vi "Application Control View.vi"(0 "Model in":refnum<class "Model.lvclass">) -> ()   [LabVIEW 2016, in "M1M3SupportEUI_Views.lvlib"]
uses:
  M1M3SupportEUI_Views.lvlib
  Model/Model.lvclass
  M1M3 Support Events/M1M3 Support Events.lvclass/M1M3 Support Events.ctl
  SALLV_m1m3/DataTypes/command_Start.ctl
  SALLV_m1m3/DataTypes/command_Standby.ctl
  SALLV_m1m3/DataTypes/command_Shutdown.ctl
  SALLV_m1m3/DataTypes/command_Enable.ctl
  SALLV_m1m3/DataTypes/command_Disable.ctl
  SALLV_m1m3/DataTypes/command_EnterEngineering.ctl
  SALLV_m1m3/DataTypes/command_ExitEngineering.ctl
  SALLV_m1m3/DataTypes/command_RaiseM1M3.ctl
  SALLV_m1m3/DataTypes/command_AbortRaiseM1M3.ctl
  SALLV_m1m3/DataTypes/command_LowerM1M3.ctl
  M1M3 Support Events/M1M3 Support Events.lvclass
  SALLV_m1m3/SALLV_m1m3.lvlib
  EUI Events/EUI Events.lvclass
panel:
  in  "AbortRaiseMirror IsTrue":bool
  in  "LowerMirror IsTrue":bool
  in  "ExitEngineering IsTrue":bool
  in  "RaiseMirror IsTrue":bool
  in  "EnterEngineering IsTrue":bool
  in  "disableIsTrue":bool
  in  "enableIsTrue":bool
  in  "standbyIsTrue":bool
  in  "shutdownIsTrue":bool
  in  "startIsTrue":bool
types:
  T1 = typedef "M1M3SupportEUI_TypeDefs.lvlib/M1M3 Support Events.ctl" = cluster{"Inclinometer  Data":refnum<user-event>, "IMS Data":refnum<user-event>, "SAL Connected":refnum<user-event>, "Accelerometer Data":refnum<user-event>, "OuterLoop Data":refnum<user-event>, "ErrorCode Event":refnum<user-event>, "InterlockStatus Event":refnum<user-event>, "InterlockWarning Event":refnum<user-event>, "Gyro Data":refnum<user-event>, "HP Actuator Info Event":refnum<user-event>, " FA Info Event":refnum<user-event>, "HP Monitor Info Event":refnum<user-event>, "FA Data":refnum<user-event>, "HP Actuator data":refnum<user-event>, "HP Monitor data":refnum<user-event>, "Air Supply Status Event":refnum<user-event>, "Air Supply Warning Event":refnum<user-event>, "Power Data":refnum<user-event>, "PID Data":refnum<user-event>, "PID Info Event":refnum<user-event>, "Power Status Event":refnum<user-event>, "Power Supply Status Event":refnum<user-event>, "Power Warning Event":refnum<user-event>, "Summary State Event":refnum<user-event>, "Detailed State Event":refnum<user-event>, "FA Force Warning Event":refnum<user-event>, "FA Warning Event":refnum<user-event>, "FA State Event":refnum<user-event>, "Applied AberrationForces Event":refnum<user-event>, "Applied Acceleration Forcces Event":refnum<user-event>, "Applied Azimuth Forces Event":refnum<user-event>, "Applied Active Optic Forces Event":refnum<user-event>, "Applied Balance Forces Event":refnum<user-event>, "Applied Cylinder Forces Event":refnum<user-event>, "Applied Elevation Forces Event":refnum<user-event>, "Applied Forces Event":refnum<user-event>, "Applied Offset Forces Event":refnum<user-event>, "Applied Static Forces Event":refnum<user-event>, "Applied Thermal Forces Event":refnum<user-event>, "Applied Velocity Forces Event":refnum<user-event>, "Rejected Aberration Force Event":refnum<user-event>, "Rejected Acceleration Forces Event":refnum<user-event>, "Rejected Active Optic Forces Event":refnum<user-event>, "Rejected Azimuth Forces Event":refnum<user-event>, "Rejected Balance Forces Event":refnum<user-event>, "Rejected Cylinder Forces Event":refnum<user-event>, "Rejected Elevation Forces Event":refnum<user-event>, "Rejected Forces Event":refnum<user-event>, "Rejected Offset Forces Event":refnum<user-event>, "Rejected Static Forces Event":refnum<user-event>, "Rejected Thermal Forces Event":refnum<user-event>, "Rejected Velocity Forces Event":refnum<user-event>, "Command Rejection Event":refnum<user-event>, "Setting Verions Event":refnum<user-event>, "Settings Applied Event":refnum<user-event>, "HP Actuator State Event":refnum<user-event>, "HP Actuator Warning Event":refnum<user-event>, "HP Monitor State Event":refnum<user-event>, "HP Monitor Warning Event":refnum<user-event>, "Accelerometer Warning Event":refnum<user-event>, "Applied Settings Match Start Event":refnum<user-event>, "Cell Light Status Event ":refnum<user-event>, "Cell Light Warning Event":refnum<user-event>, "Displacement Sensor Warning Event":refnum<user-event>, "Force Setpoint Warning Event":refnum<user-event>, "Gyro Warning Event ":refnum<user-event>, "ILC Warning Event ":refnum<user-event>, "Inclinometer Sensor Warning Event ":refnum<user-event>}
  T2 = enum16{"", "DetailedState_DetailedStates_DisabledState", "DetailedState_DetailedStates_EnabledState", "DetailedState_DetailedStates_FaultState", "DetailedState_DetailedStates_OfflineState", "DetailedState_DetailedStates_StandbyState", "DetailedState_DetailedStates_ParkedState", "DetailedState_DetailedStates_RaisingState", "DetailedState_DetailedStates_ActiveState", "DetailedState_DetailedStates_LoweringState", "DetailedState_DetailedStates_EngineeringState", "DetailedState_DetailedStates_ParkedEngineeringState", "DetailedState_DetailedStates_RaisingEngineeringState", "DetailedState_DetailedStates_ActiveEngineeringState", "DetailedState_DetailedStates_LoweringEngineeringState", "DetailedState_DetailedStates_LoweringFaultState", "DetailedState_DetailedStates_ProfileHardpointCorrectionState"}
  T3 = typedef "SALLV_m1m3.lvlib/command_Start.ctl" = cluster{"Start":bool, "SettingsToApply":string}
  T4 = typedef "SALLV_m1m3.lvlib/command_Standby.ctl" = cluster{"Standby":bool}
  T5 = typedef "SALLV_m1m3.lvlib/command_Shutdown.ctl" = cluster{"Shutdown":bool}
  T6 = typedef "SALLV_m1m3.lvlib/command_Enable.ctl" = cluster{"Enable":bool}
  T7 = typedef "SALLV_m1m3.lvlib/command_Disable.ctl" = cluster{"Disable":bool}
  T8 = typedef "SALLV_m1m3.lvlib/command_EnterEngineering.ctl" = cluster{"EnterEngineering":bool}
  T9 = typedef "SALLV_m1m3.lvlib/command_ExitEngineering.ctl" = cluster{"ExitEngineering":bool}
  T10 = typedef "SALLV_m1m3.lvlib/command_RaiseM1M3.ctl" = cluster{"RaiseM1M3":bool, "BypassReferencePosition":bool}
  T11 = typedef "SALLV_m1m3.lvlib/command_AbortRaiseM1M3.ctl" = cluster{"AbortRaiseM1M3":bool}
  T12 = typedef "SALLV_m1m3.lvlib/command_LowerM1M3.ctl" = cluster{"LowerM1M3":bool}
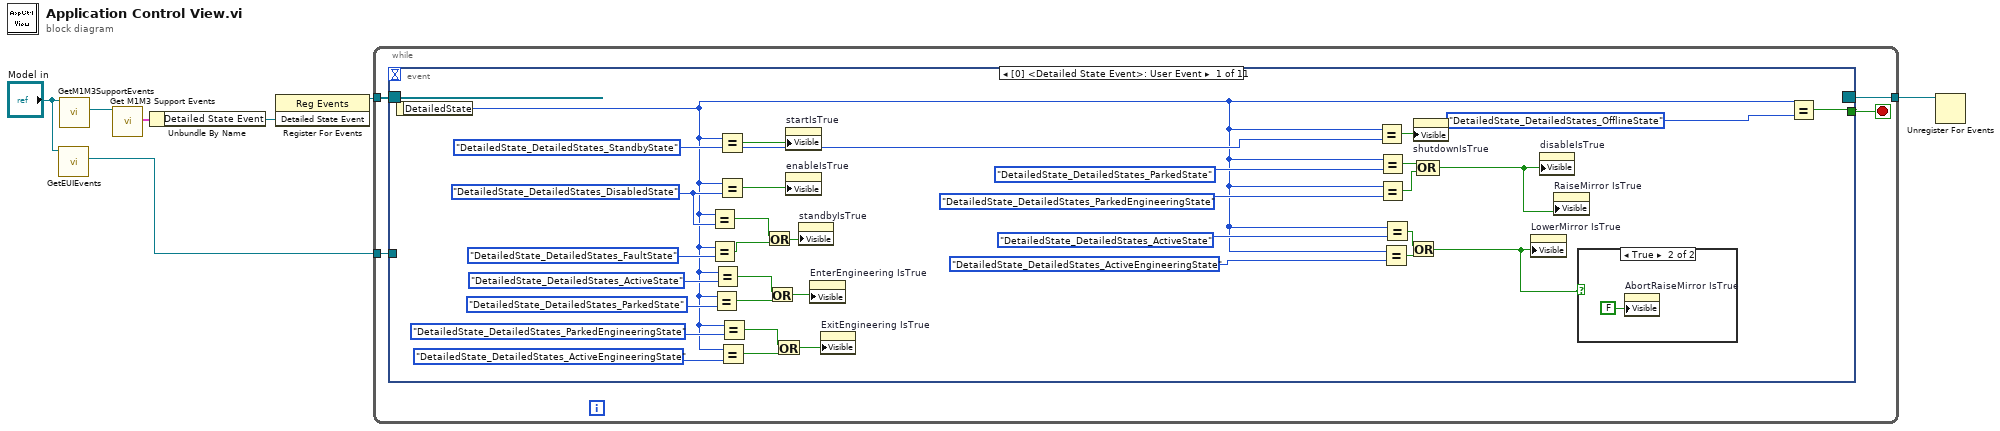
[diagram p0: block diagram]
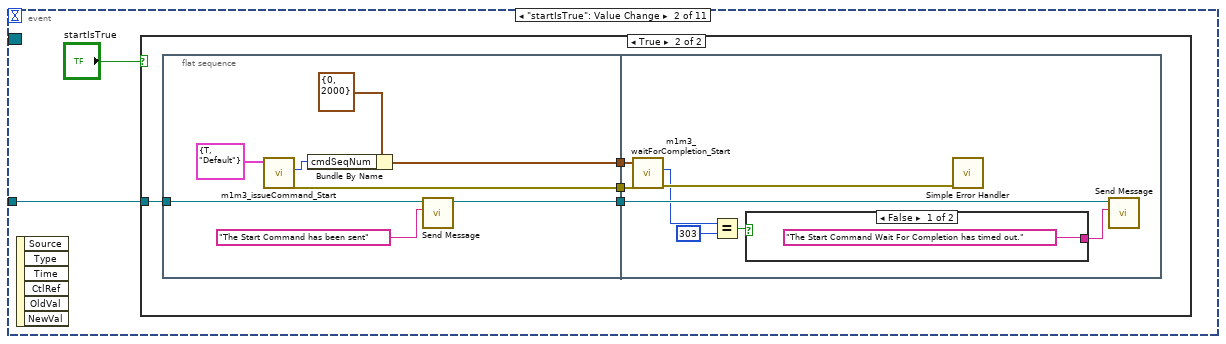
[diagram p3: hidden frame]
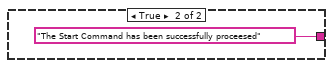
[diagram p5: hidden frame]
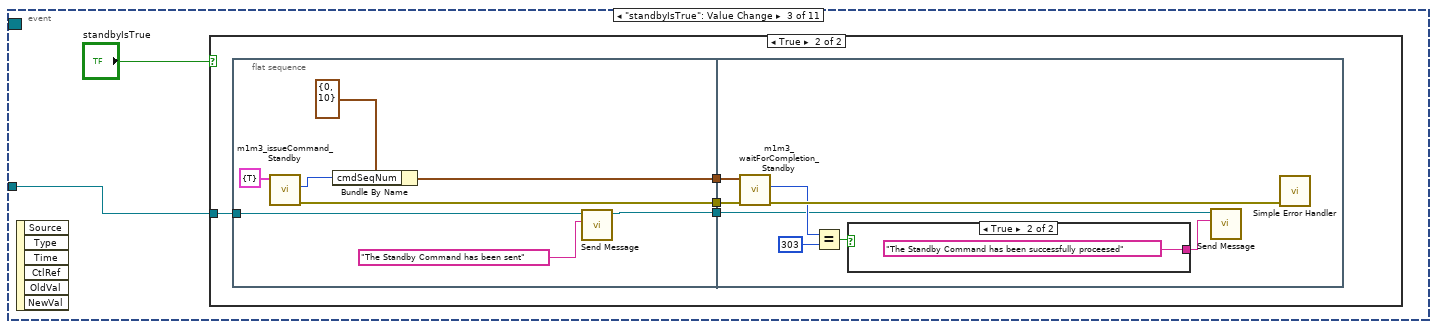
[diagram p6: hidden frame]
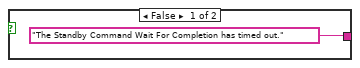
[diagram p8: hidden frame]
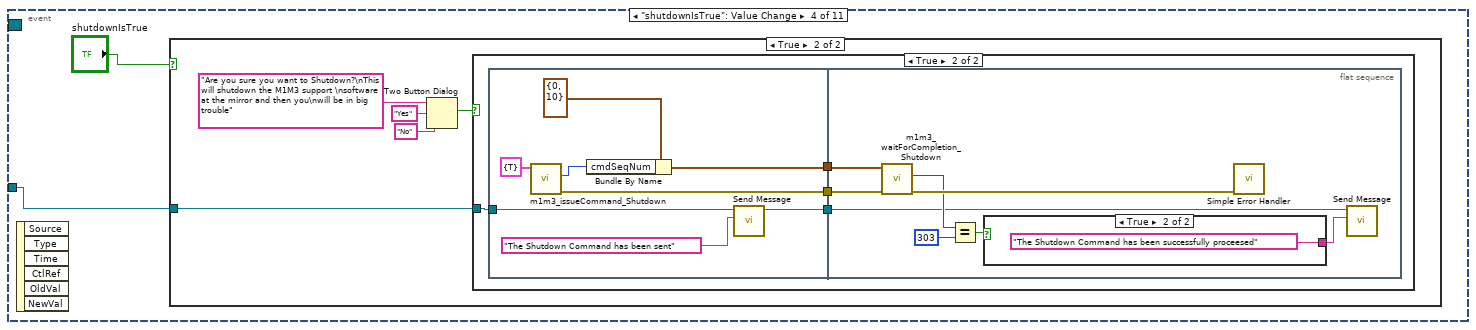
[diagram p9: hidden frame]
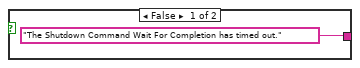
[diagram p12: hidden frame]
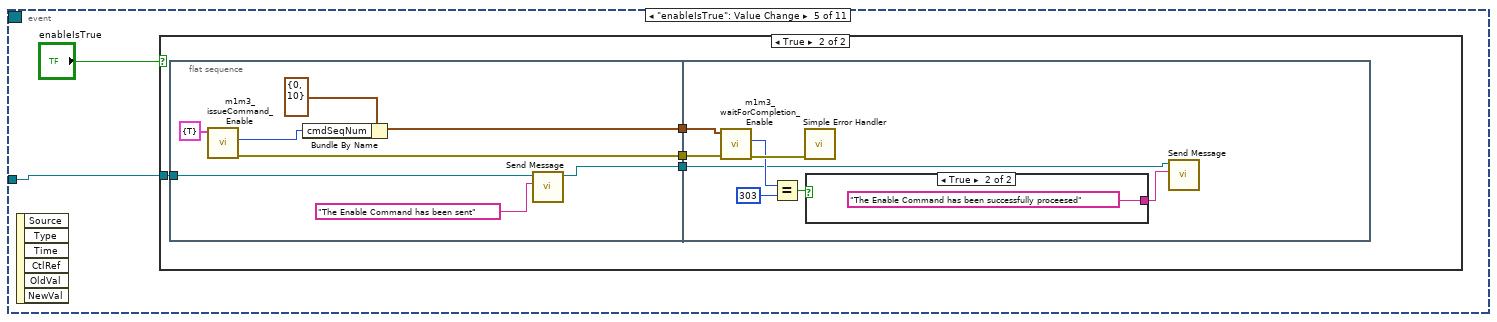
[diagram p13: hidden frame]
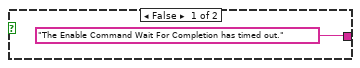
[diagram p15: hidden frame]
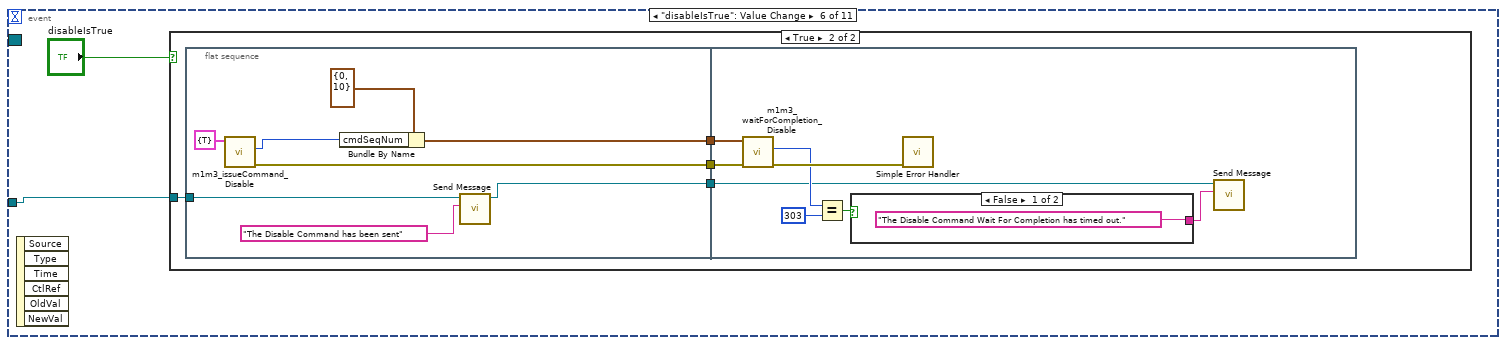
[diagram p16: hidden frame]
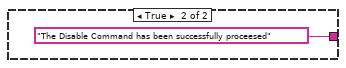
[diagram p18: hidden frame]
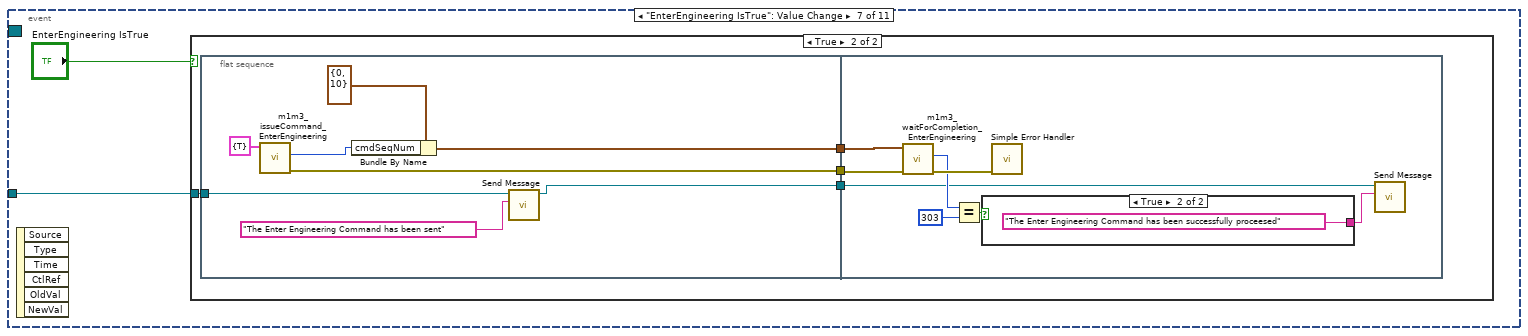
[diagram p19: hidden frame]
diagram:
  n1 = call "GetEUIEvents.vi"("Model in"="Model in") -> ("EUI Events out"=w1:refnum<class "EUI Events.lvclass">)  [unwired: 8 in, 2 out]
  n2 = call "GetM1M3SupportEvents.vi"("Model in"="Model in") -> ("M1M3 Support Events out"=w3:refnum<class "M1M3 Support Events.lvclass">)  [unwired: 8 in, 2 out]
  n3 = call "Get M1M3 Support Events.vi"("M1M3 Support Events in"=w3) -> ("M1M3 Support Events"=w6:T1)  [unwired: 9 in, 1 out]
  n4 = Unbundle By Name(w6) -> ("Detailed State Event"=w5:refnum<user-event>)
  n5 = register-events(w5) -> (reference out=w7:refnum<event-registration>)  [unwired: 2 in, 1 out]
  n6 = while {
    tunnel: w7 -> [w11]
    tunnel: [w10] -> w4
    tunnel: w1 -> [w8]
    stop <- w9 stop-if-true
    n7 = event shown="[0] <Detailed State Event>: User Event" {
      selector: w11 -> [_ _ _ _ _ _ _ _ _ _ _]
      dyn-events: [_ _ _ _ _ _ _ _ _ _ _] -> w10
      timeout: _ -> [_ _ _ _ _ _ _ _ _ _ _]
      tunnel: [w43 _ _ _ _ _ _ _ _ _ _] -> w9
      tunnel: w8 -> [_ w45 w69 w93 w122 w146 w170 w194 w218 w243 w267]
      event User Event {
        w26 = T2."DetailedState_DetailedStates_DisabledState" ("y")
        w20 = T2."DetailedState_DetailedStates_StandbyState" ("y")
        n8 = event-data() -> ("DetailedState"=w13:T2)  [unwired: 1 in]
        n9 = Equal?(x=w13, y=w26) -> (x = y?=w39:bool)
        n10 = Equal?(x=w13, y=T2."DetailedState_DetailedStates_FaultState") -> (x = y?=w40:bool)
        n11 = Equal?(x=w13, y=T2."DetailedState_DetailedStates_ParkedState") -> (x = y?=w35:bool)
        n12 = Equal?(x=w13, y=T2."DetailedState_DetailedStates_ActiveState") -> (x = y?=w36:bool)
        n13 = Equal?(x=w13, y=w20) -> (x = y?=w42:bool)
        n14 = Equal?(x=w13, y=w26) -> (x = y?=w41:bool)
        n15 = Equal?(x=w13, y=T2."DetailedState_DetailedStates_ActiveEngineeringState") -> (x = y?=w33:bool)
        n16 = Equal?(x=w13, y=T2."DetailedState_DetailedStates_ParkedEngineeringState") -> (x = y?=w32:bool)
        n17 = Or(x=w39, y=w40) -> (x .or. y?=w38:bool)
        n18 = Or(x=w36, y=w35) -> (x .or. y?=w34:bool)
        n19 = Or(x=w32, y=w33) -> (x .or. y?=w31:bool)
        n20 = property on="startIsTrue" class="Bool"("Visible"=w42) -> ()  [unwired: 2 in, 2 out]
        n21 = property on="enableIsTrue" class="Bool"("Visible"=w41) -> ()  [unwired: 2 in, 2 out]
        n22 = property on="standbyIsTrue" class="Bool"("Visible"=w38) -> ()  [unwired: 2 in, 2 out]
        n23 = property on="EnterEngineering IsTrue" class="Bool"("Visible"=w34) -> ()  [unwired: 2 in, 2 out]
        n24 = property on="ExitEngineering IsTrue" class="Bool"("Visible"=w31) -> ()  [unwired: 2 in, 2 out]
        n25 = Equal?(x=w13, y=w20) -> (x = y?=w37:bool)
        n26 = Equal?(x=w13, y=T2."DetailedState_DetailedStates_ParkedState") -> (x = y?=w28:bool)
        n27 = Equal?(x=w13, y=T2."DetailedState_DetailedStates_ParkedEngineeringState") -> (x = y?=w27:bool)
        n28 = Equal?(x=w13, y=T2."DetailedState_DetailedStates_ActiveEngineeringState") -> (x = y?=w29:bool)
        n29 = Equal?(x=w13, y=T2."DetailedState_DetailedStates_ActiveState") -> (x = y?=w30:bool)
        n30 = Or(x=w30, y=w29) -> (x .or. y?=w12:bool)
        n31 = property on="shutdownIsTrue" class="Bool"("Visible"=w37) -> ()  [unwired: 2 in, 2 out]
        n32 = Compound Arithmetic op=OR(w28, w27) -> (w17:bool)
        n33 = property on="LowerMirror IsTrue" class="Bool"("Visible"=w12) -> ()  [unwired: 2 in, 2 out]
        n34 = property on="disableIsTrue" class="Bool"("Visible"=w17) -> ()  [unwired: 2 in, 2 out]
        n35 = property on="RaiseMirror IsTrue" class="Bool"("Visible"=w17) -> ()  [unwired: 2 in, 2 out]
        n36 = case shown="True" w12 {
          frame False {
          }
          frame True {
            n37 = property on="AbortRaiseMirror IsTrue" class="Bool"("Visible"=FALSE) -> ()  [unwired: 2 in, 2 out]
          }
        }
        n38 = Equal?(x=w13, y=T2."DetailedState_DetailedStates_OfflineState") -> (x = y?=w43:bool)
      }
      event "startIsTrue": Value Change {
        n39 = event-data() -> ()  [unwired: 1 in, 6 out]
        n40 = case shown="True" "startIsTrue" {
          tunnel: w45 -> [_ w48]
          frame False {
          }
          frame True {
            n41 = flat-sequence {
              tunnel: [w57] -> w50
              tunnel: [w54] -> w49
              tunnel: w48 -> [w53]
              tunnel: [w51] -> w47
              tunnel: w50 -> [w65]
              tunnel: w49 -> [w66]
              tunnel: w47 -> [w63]
              frame #0 {
                n42 = call "m1m3_issueCommand_Start.vi"("command_Start_Ctl"=T3 {"Start"=TRUE, "SettingsToApply"="Default"}) -> ("error out"=w57:errorcluster, "function return"=w55:i32)  [unwired: 8 in, 1 out]
                n43 = Bundle By Name(cluster=cluster{"cmdSeqNum":i32, "timeout":u32} {"cmdSeqNum"=0, "timeout"=2000} ("waitComplete_Ctl"), "cmdSeqNum"=w55) -> (w54:cluster{"cmdSeqNum":i32, "timeout":u32})
                n44 = call "Send Message.vi"("Message"="The Start Command has been sent", "EUI Events in"=w53) -> ("EUI Events out"=w51:refnum<class "EUI Events.lvclass">)  [unwired: 8 in, 1 out]
              }
              frame #1 {
                n45 = call "m1m3_waitForCompletion_Start.vi"("error in (no error)"=w65, "waitComplete_Ctl"=w66) -> ("error out"=w64:errorcluster, "function return"=w61:i32)  [unwired: 7 in, 1 out]
                n46 = Equal?(x=w61, y=303) -> (x = y?=w62:bool)
                n47 = case shown="False" w62 {
                  tunnel: ["The Start Command Wait For Completion has timed out." ("Message") "The Start Command has been successfully proceesed" ("Message")] -> w60
                  frame False {
                  }
                  frame True {
                  }
                }
                n48 = call <vilib>:"Simple Error Handler.vi"("error in (no error)"=w64) -> ()  [unwired: 4 in, 5 out]
                n49 = call "Send Message.vi"("Message"=w60, "EUI Events in"=w63) -> ()  [unwired: 8 in, 2 out]
              }
            }
          }
        }
      }
      event "standbyIsTrue": Value Change {
        n50 = event-data() -> ()  [unwired: 1 in, 6 out]
        n51 = case shown="True" "standbyIsTrue" {
          tunnel: w69 -> [_ w74]
          frame False {
          }
          frame True {
            n52 = flat-sequence {
              tunnel: w74 -> [w76]
              tunnel: [w81] -> w73
              tunnel: [w78] -> w72
              tunnel: [w75] -> w71
              tunnel: w73 -> [w88]
              tunnel: w72 -> [w89]
              tunnel: w71 -> [w83]
              frame #0 {
                n53 = call "m1m3_issueCommand_Standby.vi"("command_Standby_Ctl"=T4 {"Standby"=TRUE}) -> ("error out"=w81:errorcluster, "function return"=w79:i32)  [unwired: 8 in, 1 out]
                n54 = Bundle By Name(cluster=cluster{"cmdSeqNum":i32, "timeout":u32} {"cmdSeqNum"=0, "timeout"=10} ("waitComplete_Ctl"), "cmdSeqNum"=w79) -> (w78:cluster{"cmdSeqNum":i32, "timeout":u32})
                n55 = call "Send Message.vi"("Message"="The Standby Command has been sent", "EUI Events in"=w76) -> ("EUI Events out"=w75:refnum<class "EUI Events.lvclass">)  [unwired: 8 in, 1 out]
              }
              frame #1 {
                n56 = call "m1m3_waitForCompletion_Standby.vi"("error in (no error)"=w88, "waitComplete_Ctl"=w89) -> ("error out"=w90:errorcluster, "function return"=w84:i32)  [unwired: 7 in, 1 out]
                n57 = Equal?(x=w84, y=303) -> (x = y?=w86:bool)
                n58 = case shown="True" w86 {
                  tunnel: ["The Standby Command Wait For Completion has timed out." ("Message") "The Standby Command has been successfully proceesed" ("Message")] -> w87
                  frame False {
                  }
                  frame True {
                  }
                }
                n59 = call "Send Message.vi"("Message"=w87, "EUI Events in"=w83) -> ()  [unwired: 8 in, 2 out]
                n60 = call <vilib>:"Simple Error Handler.vi"("error in (no error)"=w90) -> ()  [unwired: 4 in, 5 out]
              }
            }
          }
        }
      }
      event "shutdownIsTrue": Value Change {
        n61 = event-data() -> ()  [unwired: 1 in, 6 out]
        n62 = case shown="True" "shutdownIsTrue" {
          tunnel: w93 -> [_ w95]
          frame False {
          }
          frame True {
            n63 = Two Button Dialog(message="Are you sure you want to Shutdown?\nThis will shutdown the M1M3 support \nsoftware at the mirror and then you\nwill be in big trouble", 1:"No" ("F button name (\"Cancel\")"), 2:"Yes" ("T button name (\"OK\")")) -> (T button?=w99:bool)
            n64 = case shown="True" w99 {
              tunnel: w95 -> [_ w101]
              frame False {
              }
              frame True {
                n65 = flat-sequence {
                  tunnel: [w108] -> w103
                  tunnel: [w107] -> w102
                  tunnel: w101 -> [w105]
                  tunnel: [w104] -> w100
                  tunnel: w103 -> [w118]
                  tunnel: w102 -> [w117]
                  tunnel: w100 -> [w112]
                  frame #0 {
                    n66 = call "m1m3_issueCommand_Shutdown.vi"("command_Shutdown_Ctl"=T5 {"Shutdown"=TRUE}) -> ("error out"=w107:errorcluster, "function return"=w110:i32)  [unwired: 8 in, 1 out]
                    n67 = Bundle By Name(cluster=cluster{"cmdSeqNum":i32, "timeout":u32} {"cmdSeqNum"=0, "timeout"=10} ("waitComplete_Ctl"), "cmdSeqNum"=w110) -> (w108:cluster{"cmdSeqNum":i32, "timeout":u32})
                    n68 = call "Send Message.vi"("Message"="The Shutdown Command has been sent", "EUI Events in"=w105) -> ("EUI Events out"=w104:refnum<class "EUI Events.lvclass">)  [unwired: 8 in, 1 out]
                  }
                  frame #1 {
                    n69 = call "m1m3_waitForCompletion_Shutdown.vi"("error in (no error)"=w117, "waitComplete_Ctl"=w118) -> ("error out"=w119:errorcluster, "function return"=w113:i32)  [unwired: 7 in, 1 out]
                    n70 = Equal?(x=w113, y=303) -> (x = y?=w115:bool)
                    n71 = case shown="True" w115 {
                      tunnel: ["The Shutdown Command Wait For Completion has timed out." ("Message") "The Shutdown Command has been successfully proceesed" ("Message")] -> w116
                      frame False {
                      }
                      frame True {
                      }
                    }
                    n72 = call <vilib>:"Simple Error Handler.vi"("error in (no error)"=w119) -> ()  [unwired: 4 in, 5 out]
                    n73 = call "Send Message.vi"("Message"=w116, "EUI Events in"=w112) -> ()  [unwired: 8 in, 2 out]
                  }
                }
              }
            }
          }
        }
      }
      event "enableIsTrue": Value Change {
        n74 = event-data() -> ()  [unwired: 1 in, 6 out]
        n75 = case shown="True" "enableIsTrue" {
          tunnel: w122 -> [_ w125]
          frame False {
          }
          frame True {
            n76 = flat-sequence {
              tunnel: [w132] -> w127
              tunnel: [w131] -> w126
              tunnel: w125 -> [w129]
              tunnel: [w128] -> w124
              tunnel: w127 -> [w142]
              tunnel: w126 -> [w141]
              tunnel: w124 -> [w136]
              frame #0 {
                n77 = call "m1m3_issueCommand_Enable.vi"("command_Enable_Ctl"=T6 {"Enable"=TRUE}) -> ("error out"=w131:errorcluster, "function return"=w133:i32)  [unwired: 8 in, 1 out]
                n78 = Bundle By Name(cluster=cluster{"cmdSeqNum":i32, "timeout":u32} {"cmdSeqNum"=0, "timeout"=10} ("waitComplete_Ctl"), "cmdSeqNum"=w133) -> (w132:cluster{"cmdSeqNum":i32, "timeout":u32})
                n79 = call "Send Message.vi"("Message"="The Enable Command has been sent", "EUI Events in"=w129) -> ("EUI Events out"=w128:refnum<class "EUI Events.lvclass">)  [unwired: 8 in, 1 out]
              }
              frame #1 {
                n80 = call "m1m3_waitForCompletion_Enable.vi"("error in (no error)"=w141, "waitComplete_Ctl"=w142) -> ("error out"=w143:errorcluster, "function return"=w137:i32)  [unwired: 7 in, 1 out]
                n81 = Equal?(x=w137, y=303) -> (x = y?=w139:bool)
                n82 = call <vilib>:"Simple Error Handler.vi"("error in (no error)"=w143) -> ()  [unwired: 4 in, 5 out]
                n83 = case shown="True" w139 {
                  tunnel: ["The Enable Command Wait For Completion has timed out." ("Message") "The Enable Command has been successfully proceesed" ("Message")] -> w140
                  frame False {
                  }
                  frame True {
                  }
                }
                n84 = call "Send Message.vi"("Message"=w140, "EUI Events in"=w136) -> ()  [unwired: 8 in, 2 out]
              }
            }
          }
        }
      }
      event "disableIsTrue": Value Change {
        n85 = event-data() -> ()  [unwired: 1 in, 6 out]
        n86 = case shown="True" "disableIsTrue" {
          tunnel: w146 -> [_ w151]
          frame False {
          }
          frame True {
            n87 = flat-sequence {
              tunnel: w151 -> [w155]
              tunnel: [w154] -> w150
              tunnel: [w153] -> w149
              tunnel: [w152] -> w148
              tunnel: w150 -> [w163]
              tunnel: w149 -> [w162]
              tunnel: w148 -> [w160]
              frame #0 {
                n88 = call "m1m3_issueCommand_Disable.vi"("command_Disable_Ctl"=T7 {"Disable"=TRUE}) -> ("error out"=w153:errorcluster, "function return"=w157:i32)  [unwired: 8 in, 1 out]
                n89 = Bundle By Name(cluster=cluster{"cmdSeqNum":i32, "timeout":u32} {"cmdSeqNum"=0, "timeout"=10} ("waitComplete_Ctl"), "cmdSeqNum"=w157) -> (w154:cluster{"cmdSeqNum":i32, "timeout":u32})
                n90 = call "Send Message.vi"("Message"="The Disable Command has been sent", "EUI Events in"=w155) -> ("EUI Events out"=w152:refnum<class "EUI Events.lvclass">)  [unwired: 8 in, 1 out]
              }
              frame #1 {
                n91 = call "m1m3_waitForCompletion_Disable.vi"("error in (no error)"=w162, "waitComplete_Ctl"=w163) -> ("error out"=w164:errorcluster, "function return"=w161:i32)  [unwired: 7 in, 1 out]
                n92 = Equal?(x=w161, y=303) -> (x = y?=w166:bool)
                n93 = case shown="False" w166 {
                  tunnel: ["The Disable Command Wait For Completion has timed out." ("Message") "The Disable Command has been successfully proceesed" ("Message")] -> w167
                  frame False {
                  }
                  frame True {
                  }
                }
                n94 = call <vilib>:"Simple Error Handler.vi"("error in (no error)"=w164) -> ()  [unwired: 4 in, 5 out]
                n95 = call "Send Message.vi"("Message"=w167, "EUI Events in"=w160) -> ()  [unwired: 8 in, 2 out]
              }
            }
          }
        }
      }
      event "EnterEngineering IsTrue": Value Change {
        n96 = event-data() -> ()  [unwired: 1 in, 6 out]
        n97 = case shown="True" "EnterEngineering IsTrue" {
          tunnel: w170 -> [_ w173]
          frame False {
          }
          frame True {
            n98 = flat-sequence {
              tunnel: [w180] -> w175
              tunnel: [w179] -> w174
              tunnel: w173 -> [w177]
              tunnel: [w176] -> w172
              tunnel: w175 -> [w190]
              tunnel: w174 -> [w189]
              tunnel: w172 -> [w184]
              frame #0 {
                n99 = call "m1m3_issueCommand_EnterEngineering.vi"("command_EnterEngineering_Ctl"=T8 {"EnterEngineering"=TRUE}) -> ("error out"=w179:errorcluster, "function return"=w181:i32)  [unwired: 8 in, 1 out]
                n100 = Bundle By Name(cluster=cluster{"cmdSeqNum":i32, "timeout":u32} {"cmdSeqNum"=0, "timeout"=10} ("waitComplete_Ctl"), "cmdSeqNum"=w181) -> (w180:cluster{"cmdSeqNum":i32, "timeout":u32})
                n101 = call "Send Message.vi"("Message"="The Enter Engineering Command has been sent", "EUI Events in"=w177) -> ("EUI Events out"=w176:refnum<class "EUI Events.lvclass">)  [unwired: 8 in, 1 out]
              }
              frame #1 {
                n102 = call "m1m3_waitForCompletion_EnterEngineering.vi"("error in (no error)"=w189, "waitComplete_Ctl"=w190) -> ("error out"=w191:errorcluster, "function return"=w185:i32)  [unwired: 7 in, 1 out]
                n103 = Equal?(x=w185, y=303) -> (x = y?=w187:bool)
                n104 = case shown="True" w187 {
                  tunnel: ["The Enter Engineering Command Wait For Completion has timed out." ("Message") "The Enter Engineering Command has been successfully proceesed" ("Message")] -> w188
                  frame False {
                  }
                  frame True {
                  }
                }
                n105 = call <vilib>:"Simple Error Handler.vi"("error in (no error)"=w191) -> ()  [unwired: 4 in, 5 out]
                n106 = call "Send Message.vi"("Message"=w188, "EUI Events in"=w184) -> ()  [unwired: 8 in, 2 out]
              }
            }
          }
        }
      }
      event "ExitEngineering IsTrue": Value Change {
        n107 = event-data() -> ()  [unwired: 1 in, 6 out]
        n108 = case shown="True" "ExitEngineering IsTrue" {
          tunnel: w194 -> [_ w197]
          frame False {
          }
          frame True {
            n109 = flat-sequence {
              tunnel: [w204] -> w199
              tunnel: [w203] -> w198
              tunnel: w197 -> [w201]
              tunnel: [w200] -> w196
              tunnel: w199 -> [w214]
              tunnel: w198 -> [w213]
              tunnel: w196 -> [w209]
              frame #0 {
                n110 = call "m1m3_issueCommand_ExitEngineering.vi"("command_ExitEngineering_Ctl"=T9 {"ExitEngineering"=TRUE}) -> ("error out"=w203:errorcluster, "function return"=w205:i32)  [unwired: 8 in, 1 out]
                n111 = Bundle By Name(cluster=cluster{"cmdSeqNum":i32, "timeout":u32} {"cmdSeqNum"=0, "timeout"=10} ("waitComplete_Ctl"), "cmdSeqNum"=w205) -> (w204:cluster{"cmdSeqNum":i32, "timeout":u32})
                n112 = call "Send Message.vi"("Message"="The Exit Engineering Command has been sent", "EUI Events in"=w201) -> ("EUI Events out"=w200:refnum<class "EUI Events.lvclass">)  [unwired: 8 in, 1 out]
              }
              frame #1 {
                n113 = call "m1m3_waitForCompletion_ExitEngineering.vi"("error in (no error)"=w213, "waitComplete_Ctl"=w214) -> ("error out"=w215:errorcluster, "function return"=w208:i32)  [unwired: 7 in, 1 out]
                n114 = Equal?(x=w208, y=303) -> (x = y?=w211:bool)
                n115 = call <vilib>:"Simple Error Handler.vi"("error in (no error)"=w215) -> ()  [unwired: 4 in, 5 out]
                n116 = case shown="True" w211 {
                  tunnel: ["The Exit Engineering Command Wait For Completion has timed out." ("Message") "The Exit Engineering Command has been successfully proceesed" ("Message")] -> w212
                  frame False {
                  }
                  frame True {
                  }
                }
                n117 = call "Send Message.vi"("Message"=w212, "EUI Events in"=w209) -> ()  [unwired: 8 in, 2 out]
              }
            }
          }
        }
      }
      event "RaiseMirror IsTrue": Value Change {
        n118 = event-data() -> ()  [unwired: 1 in, 6 out]
        n119 = case shown="True" "RaiseMirror IsTrue" {
          tunnel: w218 -> [_ w223]
          frame False {
          }
          frame True {
            n120 = flat-sequence {
              tunnel: w223 -> [w227]
              tunnel: [w226] -> w222
              tunnel: [w225] -> w221
              tunnel: [w224] -> w220
              tunnel: w222 -> [w237]
              tunnel: w221 -> [w235]
              tunnel: w220 -> [w234]
              frame #0 {
                n121 = call "m1m3_issueCommand_RaiseM1M3.vi"("command_RaiseM1M3_Ctl"=T10 {"RaiseM1M3"=TRUE, "BypassReferencePosition"=FALSE}) -> ("error out"=w224:errorcluster, "function return"=w230:i32)  [unwired: 8 in, 1 out]
                n122 = Bundle By Name(cluster=cluster{"cmdSeqNum":i32, "timeout":u32} {"cmdSeqNum"=0, "timeout"=10} ("waitComplete_Ctl"), "cmdSeqNum"=w230) -> (w225:cluster{"cmdSeqNum":i32, "timeout":u32})
                n123 = property on="AbortRaiseMirror IsTrue" class="Bool"("Visible"=TRUE) -> ()  [unwired: 2 in, 2 out]
                n124 = call "Send Message.vi"("Message"="The Raise Mirror Command has been sent", "EUI Events in"=w227) -> ("EUI Events out"=w226:refnum<class "EUI Events.lvclass">)  [unwired: 8 in, 1 out]
              }
              frame #1 {
                n125 = call "m1m3_waitForCompletion_RaiseM1M3.vi"("error in (no error)"=w234, "waitComplete_Ctl"=w235) -> ("error out"=w236:errorcluster, "function return"=w233:i32)  [unwired: 7 in, 1 out]
                n126 = Equal?(x=w233, y=303) -> (x = y?=w239:bool)
                n127 = case shown="False" w239 {
                  tunnel: ["The Raise Mirror Command Wait For Completion has timed out." ("Message") "The Raise Mirror Command has been successfully proceesed" ("Message")] -> w240
                  frame False {
                  }
                  frame True {
                  }
                }
                n128 = call <vilib>:"Simple Error Handler.vi"("error in (no error)"=w236) -> ()  [unwired: 4 in, 5 out]
                n129 = call "Send Message.vi"("Message"=w240, "EUI Events in"=w237) -> ()  [unwired: 8 in, 2 out]
              }
            }
          }
        }
      }
      event "AbortRaiseMirror IsTrue": Value Change {
        n130 = event-data() -> ()  [unwired: 1 in, 6 out]
        n131 = case shown="True" "AbortRaiseMirror IsTrue" {
          tunnel: w243 -> [_ w246]
          frame False {
          }
          frame True {
            n132 = flat-sequence {
              tunnel: [w253] -> w248
              tunnel: [w252] -> w247
              tunnel: w246 -> [w250]
              tunnel: [w249] -> w245
              tunnel: w248 -> [w263]
              tunnel: w247 -> [w262]
              tunnel: w245 -> [w258]
              frame #0 {
                n133 = call "m1m3_issueCommand_AbortRaiseM1M3.vi"("command_AbortRaiseM1M3_Ctl"=T11 {"AbortRaiseM1M3"=TRUE}) -> ("error out"=w252:errorcluster, "function return"=w254:i32)  [unwired: 8 in, 1 out]
                n134 = Bundle By Name(cluster=cluster{"cmdSeqNum":i32, "timeout":u32} {"cmdSeqNum"=0, "timeout"=10} ("waitComplete_Ctl"), "cmdSeqNum"=w254) -> (w253:cluster{"cmdSeqNum":i32, "timeout":u32})
                n135 = call "Send Message.vi"("Message"="The Abort Raise Mirror Command has been sent", "EUI Events in"=w250) -> ("EUI Events out"=w249:refnum<class "EUI Events.lvclass">)  [unwired: 8 in, 1 out]
              }
              frame #1 {
                n136 = call "m1m3_waitForCompletion_AbortRaiseM1M3.vi"("error in (no error)"=w262, "waitComplete_Ctl"=w263) -> ("error out"=w264:errorcluster, "function return"=w257:i32)  [unwired: 7 in, 1 out]
                n137 = Equal?(x=w257, y=303) -> (x = y?=w260:bool)
                n138 = call <vilib>:"Simple Error Handler.vi"("error in (no error)"=w264) -> ()  [unwired: 4 in, 5 out]
                n139 = case shown="True" w260 {
                  tunnel: ["The Abort Raise Mirror Command Wait For Completion has timed out." ("Message") "The Abort Raise Mirror Command has been successfully proceesed" ("Message")] -> w261
                  frame False {
                  }
                  frame True {
                  }
                }
                n140 = call "Send Message.vi"("Message"=w261, "EUI Events in"=w258) -> ()  [unwired: 8 in, 2 out]
              }
            }
          }
        }
      }
      event "LowerMirror IsTrue": Value Change {
        n141 = event-data() -> ()  [unwired: 1 in, 6 out]
        n142 = case shown="True" "LowerMirror IsTrue" {
          tunnel: w267 -> [_ w272]
          frame False {
          }
          frame True {
            n143 = flat-sequence {
              tunnel: w272 -> [w276]
              tunnel: [w275] -> w271
              tunnel: [w274] -> w270
              tunnel: [w273] -> w269
              tunnel: w271 -> [w285]
              tunnel: w270 -> [w283]
              tunnel: w269 -> [w282]
              frame #0 {
                n144 = call "m1m3_issueCommand_LowerM1M3.vi"("command_LowerM1M3_Ctl"=T12 {"LowerM1M3"=TRUE}) -> ("error out"=w273:errorcluster, "function return"=w278:i32)  [unwired: 8 in, 1 out]
                n145 = Bundle By Name(cluster=cluster{"cmdSeqNum":i32, "timeout":u32} {"cmdSeqNum"=0, "timeout"=10} ("waitComplete_Ctl"), "cmdSeqNum"=w278) -> (w274:cluster{"cmdSeqNum":i32, "timeout":u32})
                n146 = call "Send Message.vi"("Message"="The Lower Mirror Command has been sent", "EUI Events in"=w276) -> ("EUI Events out"=w275:refnum<class "EUI Events.lvclass">)  [unwired: 8 in, 1 out]
              }
              frame #1 {
                n147 = call "m1m3_waitForCompletion_LowerM1M3.vi"("error in (no error)"=w282, "waitComplete_Ctl"=w283) -> ("error out"=w284:errorcluster, "function return"=w281:i32)  [unwired: 7 in, 1 out]
                n148 = Equal?(x=w281, y=303) -> (x = y?=w287:bool)
                n149 = call <vilib>:"Simple Error Handler.vi"("error in (no error)"=w284) -> ()  [unwired: 4 in, 5 out]
                n150 = case shown="True" w287 {
                  tunnel: ["The Lower Mirror Command Wait For Completion has timed out." ("Message") "The Lower Mirror Command has been successfully proceesed" ("Message")] -> w288
                  frame False {
                  }
                  frame True {
                  }
                }
                n151 = call "Send Message.vi"("Message"=w288, "EUI Events in"=w285) -> ()  [unwired: 8 in, 2 out]
              }
            }
          }
        }
      }
    }
  }
  n152 = Unregister For Events(event registration refnum=w4) -> ()  [unwired: 1 in, 1 out]
